vi "Data Output Format.vi"(5 "Byte Order (Normal)":T1(ring), 7 "ASCII Precision (6)":i32=6 min=1 max=16, 8 "error in (no error)":errorcluster, 9 "Data Format (ASCII)":T2(ring), 10 "Node In":string, 11 "VISA resource name":refnum<visa-resource-name>) -> (0 "error out":errorcluster, 2 "Node Out":string, 3 "VISA resource name out":refnum<visa-resource-name>, 4 "Command String":string)   [LabVIEW 2017, in "Keithley 2600 Series.lvlib"]
doc: "This VI configures the data output format used by the printnumber() and printbuffer() functions."
uses:
  Keithley 2600 Series.lvlib
  Private/GlobalVariables.vi
panel:
  # "(c) 2008 Keithley Instruments, Inc.  ALL RIGHTS RESERVED."
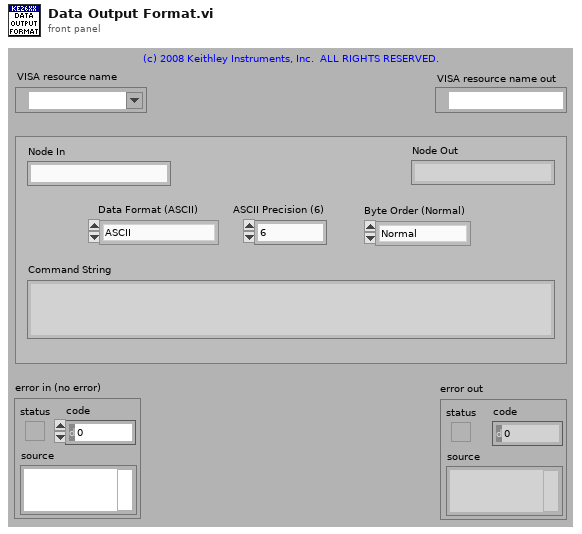
[diagram p1: front panel]
types:
  T1 = enum32{"Normal", "Big Endian", "Little Endian", "Network", "Swapped"}
  T2 = enum32{"ASCII", "Real 32", "Real 64", "Single Precision Real", "Double Precision Real"}
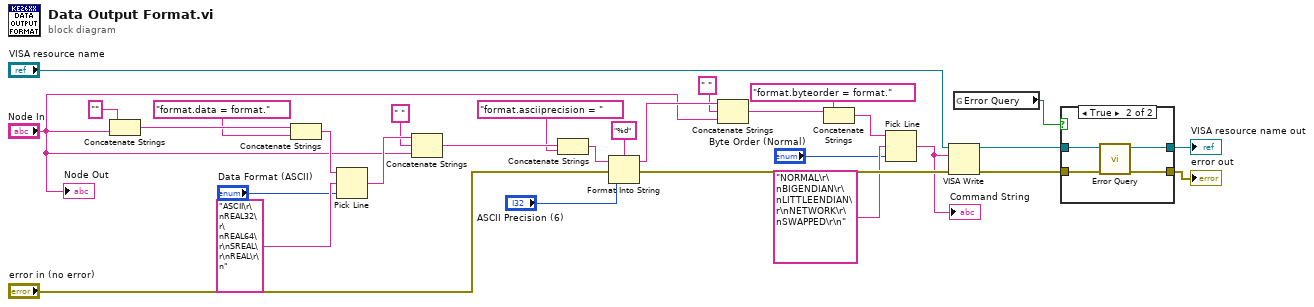
[diagram p0: block diagram]
diagram:
  n1 = Concatenate Strings("" ("command"), "Node In") -> (w29:string)
  n2 = Concatenate Strings(w29, "format.data = format." ("command")) -> (w26:string)
  n3 = Pick Line(string ("")=w26, multi-line string="ASCII\r\nREAL32\r\nREAL64\r\nSREAL\r\nREAL\r\n" ("options"), line index="Data Format (ASCII)") -> (output string=w24:string)
  n4 = Concatenate Strings(w24, " " ("command"), "Node In") -> (w21:string)
  n5 = Concatenate Strings(w21, "format.asciiprecision = " ("command")) -> (w15:string)
  n6 = Format Into String(format string="%d", initial string=w15, error in="error in (no error)", "ASCII Precision (6)") -> (resulting string=w17:string, error out=w18:errorcluster)
  n7 = Concatenate Strings(w17, " " ("command"), "Node In") -> (w12:string)
  n8 = Concatenate Strings(w12, "format.byteorder = format." ("command")) -> (w10:string)
  n9 = Pick Line(string ("")=w10, multi-line string="NORMAL\r\nBIGENDIAN\r\nLITTLEENDIAN\r\nNETWORK\r\nSWAPPED\r\n" ("options"), line index="Byte Order (Normal)") -> (output string=w6:string)
  "Command String" <- w6
  n10 = VISA Write(VISA resource name="VISA resource name", write buffer=w6, error in (no error)=w18) -> (VISA resource name out=w4:refnum<visa-resource-name>, error out=w3:errorcluster)  [unwired: 1 out]
  n11 = global read "GlobalVariables.vi" "Error Query"() -> (w5:bool)
  n12 = case shown="True" w5 {
    tunnel: w4 -> [w32 w36]
    tunnel: w3 -> [w31 w35]
    tunnel: [w32 w34] -> w2
    tunnel: [w31 w33] -> w1
    frame False {
    }
    frame True {
      n13 = call "Error Query.vi"("error in (no error)"=w35, "VISA resource name"=w36) -> ("error out"=w33:errorcluster, "VISA resource name out"=w34:refnum<visa-resource-name>)  [unwired: 8 out]
    }
  }
  "VISA resource name out" <- w2
  "error out" <- w1
  "Node Out" <- "Node In"
